vi "MasterAquisitionFile_2P.vi"() -> ()   [LabVIEW 2020]
uses:
  <vilib>/userDefined/High Color/IMAQdx.ctl
  <vilib>/vision/driver/IMAQdx.llb/IMAQdx Camera Control Mode.ctl
  <vilib>/vision/driver/IMAQdx.llb/IMAQdx Acquisition Mode.ctl
  <vilib>/vision/driver/IMAQdx.llb/IMAQdx Buffer Number Mode.ctl
  <vilib>/DAQmx/write.llb/DAQmx Write (Digital 1D Wfm NChan NSamp).vi
  <vilib>/DAQmx/read.llb/DAQmx Read (Digital 1D Bool 1Chan 1Samp).vi
  <vilib>/DAQmx/read.llb/DAQmx Read (Analog 1D Wfm NChan NSamp).vi
  <vilib>/Waveform/DWDTOps.llb/DWDT Digital to Boolean Array.vi
  <vilib>/DAQmx/create/channels.llb/DAQmx Create Channel (DO-Digital Output).vi
  <vilib>/DAQmx/configure/timing.llb/DAQmx Timing (Sample Clock).vi
  <vilib>/Waveform/DWDTOps.llb/DWDT Boolean Array to Digital.vi
  <vilib>/Waveform/DWDTOps.llb/DWDT Uncompress Digital.vi
  <vilib>/DAQmx/miscellaneous.llb/DAQmx Fill In Error Info.vi
  <vilib>/DAQmx/create/channels.llb/DAQmx Create Channel (DI-Digital Input).vi
  <vilib>/DAQmx/create/channels.llb/DAQmx Create Channel (CO-Pulse Generation-Frequency).vi
  <vilib>/DAQmx/configure/timing.llb/DAQmx Timing (Implicit).vi
  <vilib>/DAQmx/create/channels.llb/DAQmx Create Channel (AI-Voltage-Basic).vi
  <vilib>/DAQmx/configure/trigger.llb/DAQmx Start Trigger (Digital Edge).vi
  <vilib>/vision/driver/NI_Vision_Acquisition_Software.lvlib
  <resource>/objmgr/imaqdx.rc
  <resource>/objmgr/daqmx.rc
panel:
  out "Analog Data 3":bool
  out "?":T1(plugin-control)
  out "?":T1(plugin-control)
  out "Analog Data 2":bool
  in  "Pupil Fs":cluster{"Pupil Fs":u16}={"Pupil Fs"=30} {"Pupil Fs" format="%0.0f"}
  out "Pupil Cam Fs":dbl(knob) scale=0.0..200.0 scale format="%#1_6g"
  out "Dropped 2":u32(slide) caption="Pupil" scale=0.0..150.0
  out "Pupil Cam":bool
  in  "Analog Input Channels":tag="Dev1/ai0:3"
  out "Auditory":bool
  out "RPad":bool
  out "LPad":bool
  in  "Sol Stim Parameters":cluster{"Fs":dbl, "Samples":dbl}
  in  "LED Stim Parameters":cluster{"Fs":dbl, "Samples":dbl}
  in  "Generate Stimuli":bool
  in  "Sol Duty Cycle (%)":dbl=50.0
  in  "Sol Freq":dbl=5.0
  in  "Sol Dur (s)":dbl=5.0
  in  "LED Duty Cycle (%)":dbl=10.0
  in  "LED Freq":dbl=10.0
  in  "LED Dur (s)":dbl=2.0
  out "Stimulus Order":digitalwaveform[](graph)
  out "Solenoid Stim":digitalwaveform(graph)={"t0"=timestamp(0 s since 1904-01-01), "dt"=5e-05, "Y"={"transitions"=[], "data"=array100000x1[100000 elements]}}
  in  "Trial Offset (s)":dbl=45.0
  in  "Interstim (s)":dbl=45.0
  in  "Right Pad":dbl=1.0
  in  "Left Pad":dbl=1.0
  in  "Auditory":dbl=1.0
  in  "LED":dbl
  in  "stop":bool
  out "?":T1(plugin-control)
  out "Behavior Cam Fs":dbl(knob) scale=0.0..200.0
  out "Behav Cam":bool
  out "Complete":bool
  out "Whisk Cam":bool
  out "Analog":bool
  out "MScan Trig":bool
  out "?":bool[](array[boolean])=[TRUE]
  out "Hexadecimal Data":u32=1 format="%x"
  out "Time Elapsed (Min)":cluster{dbl, dbl}(slide)={1.0, 0.0} scale=0.0..16.0 scale format="%#_2g"
  out "Whisker Camera":bool
  out "Analog Data":bool
  out "Analog Samples":i32
  in  "Device Analog Channel Labels":string[](array[string])=["forceSensor", "LPadSol", "RPadSol", "AudSol", "", "", "", ""]
  in  "?":cluster{"Analog Fs":u16}={"Analog Fs"=20000} {"Analog Fs" format="%0.0f"}
  in  "?":cluster{"WhiskerCam Fs":u16}={"WhiskerCam Fs"=150}
  out "Notes Size":i32=7
  out "Notes Reversed":string[](array[string])=["Experimenter", "Animal ID", "Isoflurane time", "Amplifier Gain", "Session ID", "Hemisphere", "Solenoid PSI"]
  out "Notes Array":string[](array[string])=["Solenoid PSI", "Hemisphere", "Session ID", "Amplifier Gain", "Isoflurane time", "Animal ID", "Experimenter"]
  in  "Notes:":T2={"Experimenter"="Kevin\n", "Animal ID"="T300", "Isoflurane time"="730", "Amplifier Gain"="10000", "Session ID"="Imaging Session One", "Hemisphere"="RH", "Solenoid PSI"="10"}
  in  "Target Path":path=path "C:/Users/klt8/Documents" caption="Final Saved File Location"
  out "Dropped":u32(slide) caption="Whisk" scale=0.0..150.0
  out "Current File Name":string="221018_11_01_39"
  in  "Time (min)":dbl(knob)=1.0 min=0.5 max=20.0 step=0.5 scale=0.0..20.0 scale format="%#_3g"
  in  "Temp Path":path=path "C:/Users/klt8/Documents/LabVIEW Temp Files" caption="Temporary File Path"
  out "Whisker Cam Fs":dbl(knob) scale=0.0..200.0 scale format="%#1_6g"
  # "Notes"
  # "Dropped Frames"
  # "LPAD"
  # "RPAD"
  # "AUD"
  # "Analog Fs"
  # "Whisker Fs"
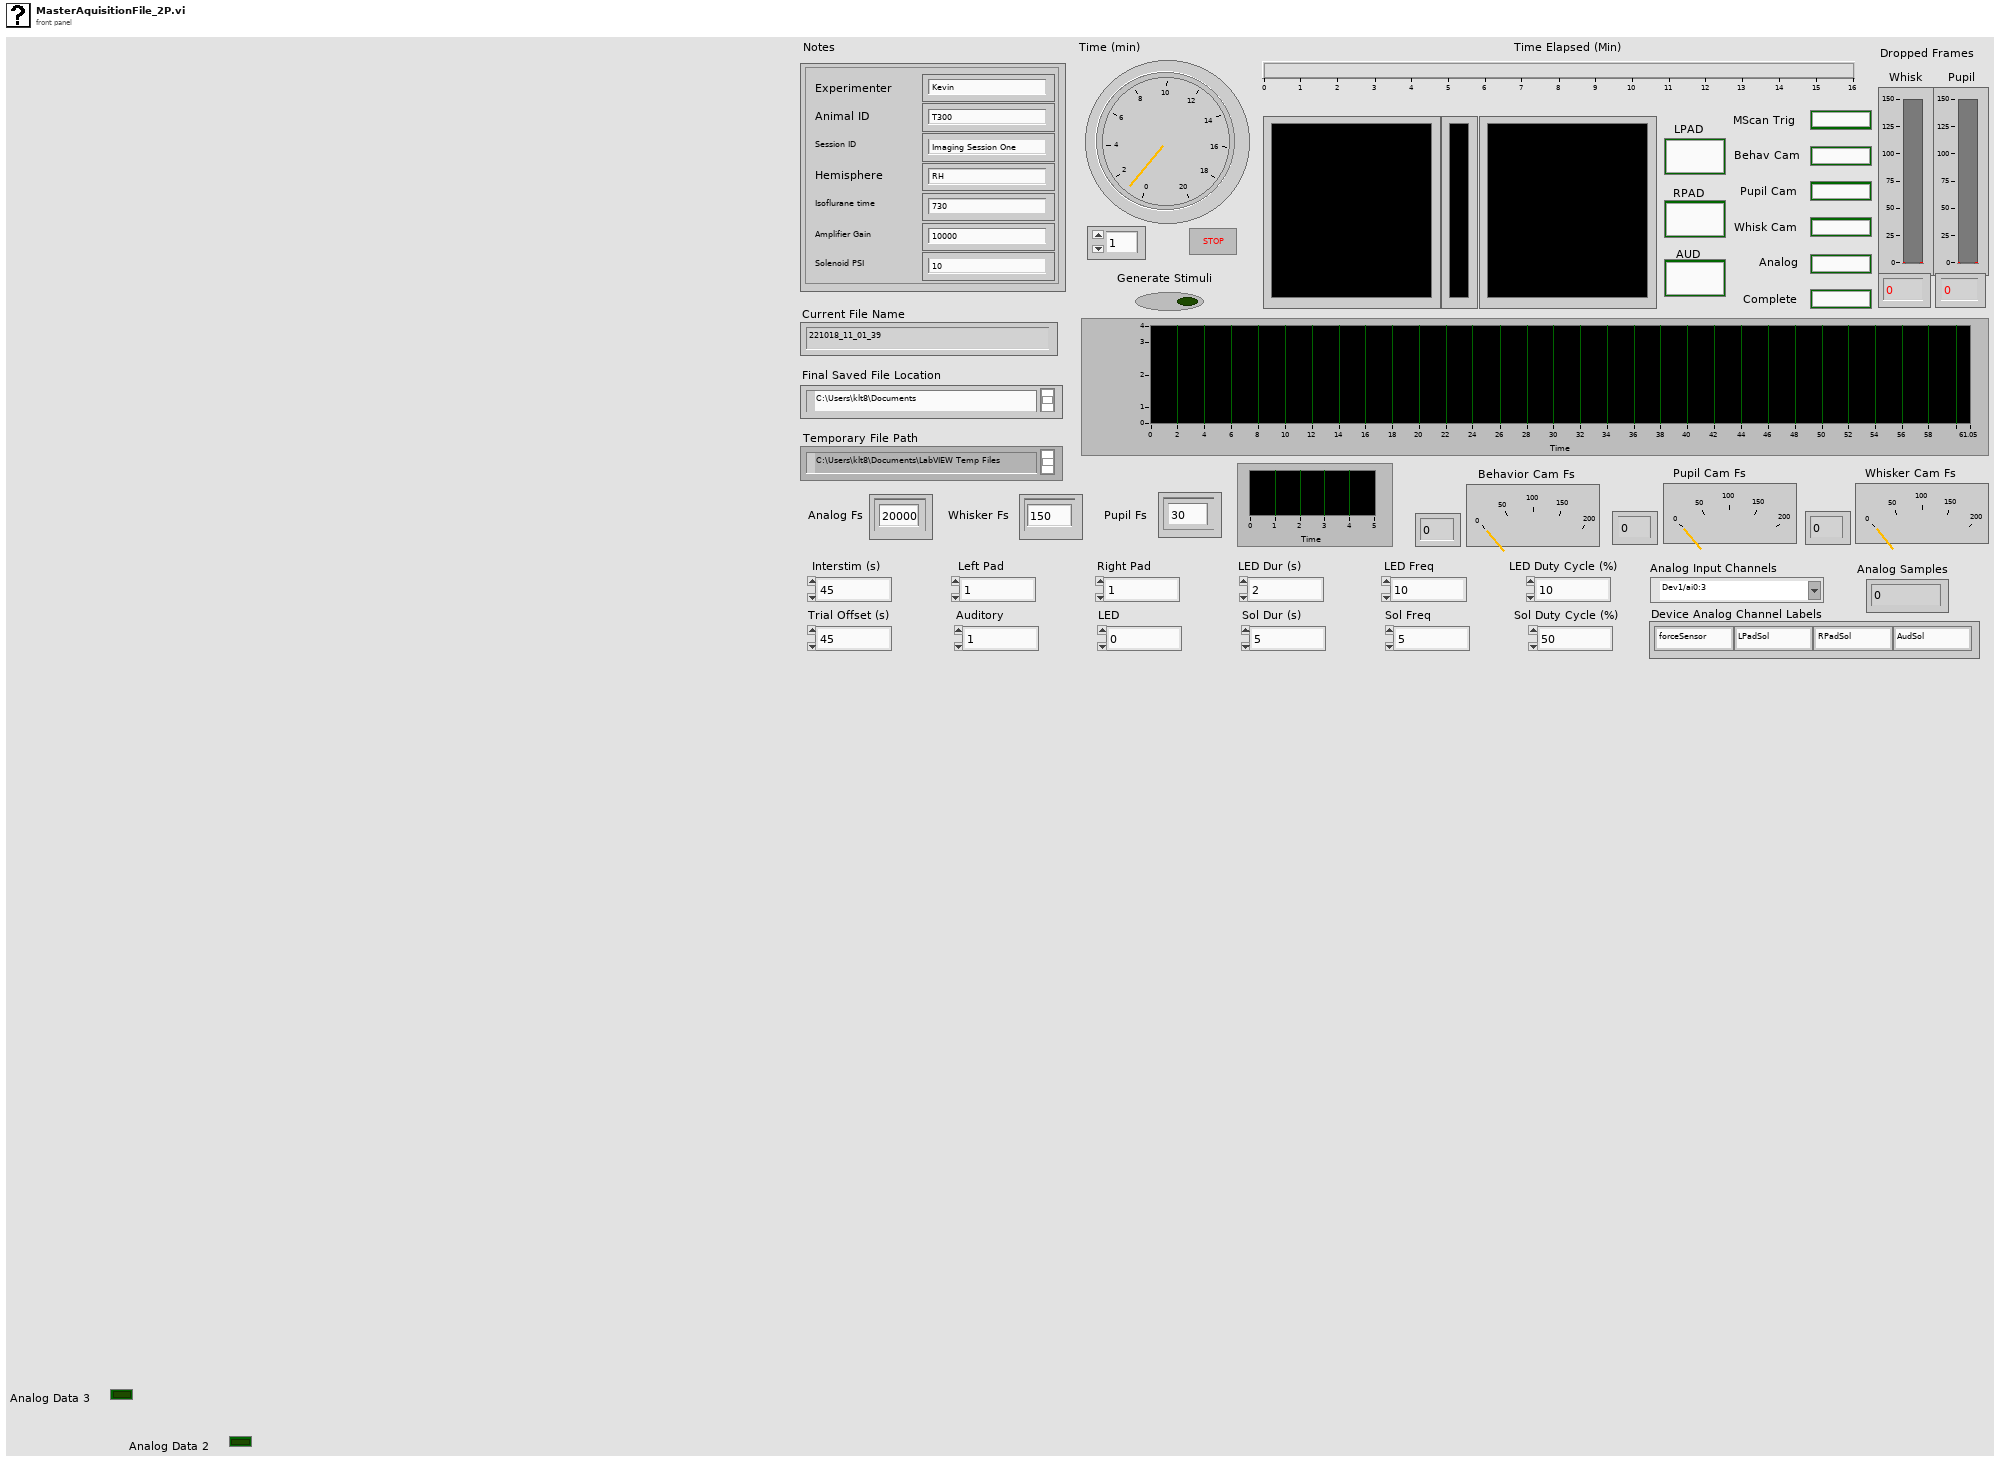
[diagram p1: front panel]
types:
  T1 = typedef "IMAQ Image.ctl" = refnum<image>
  T2 = cluster{"Experimenter":string, "Animal ID":string, "Isoflurane time":string, "Amplifier Gain":string, "Session ID":string, "Hemisphere":string, "Solenoid PSI":string}
  T3 = typedef "IMAQdx.ctl" = refnum<k21>
  T4 = enum16{"open", "replace", "create", "open or create", "replace or create", "replace or create with confirmation"}
  T5 = typedef "NI_Vision_Acquisition_Software.lvlib/IMAQdx Acquisition Mode.ctl" = enum32{"One Shot", "Continuous"}
  T6 = typedef "NI_Vision_Acquisition_Software.lvlib/IMAQdx Camera Control Mode.ctl" = enum32{"Controller", "Listener"}
  T7 = enum16{"open", "open or create", "create or replace", "create", "open (read-only)"}
  T8 = enum16{"big-endian, network order", "native, host order", "little-endian"}
  T9 = typedef "NI_Vision_Acquisition_Software.lvlib/IMAQdx Buffer Number Mode.ctl" = enum32{"Next", "Last", "Buffer Number", "Every", "Last New"}
  T10 = typedef "Image Type" = u32
  T11 = typedef "IMAQ AVI2 Refnum.ctl" = refnum<k20>
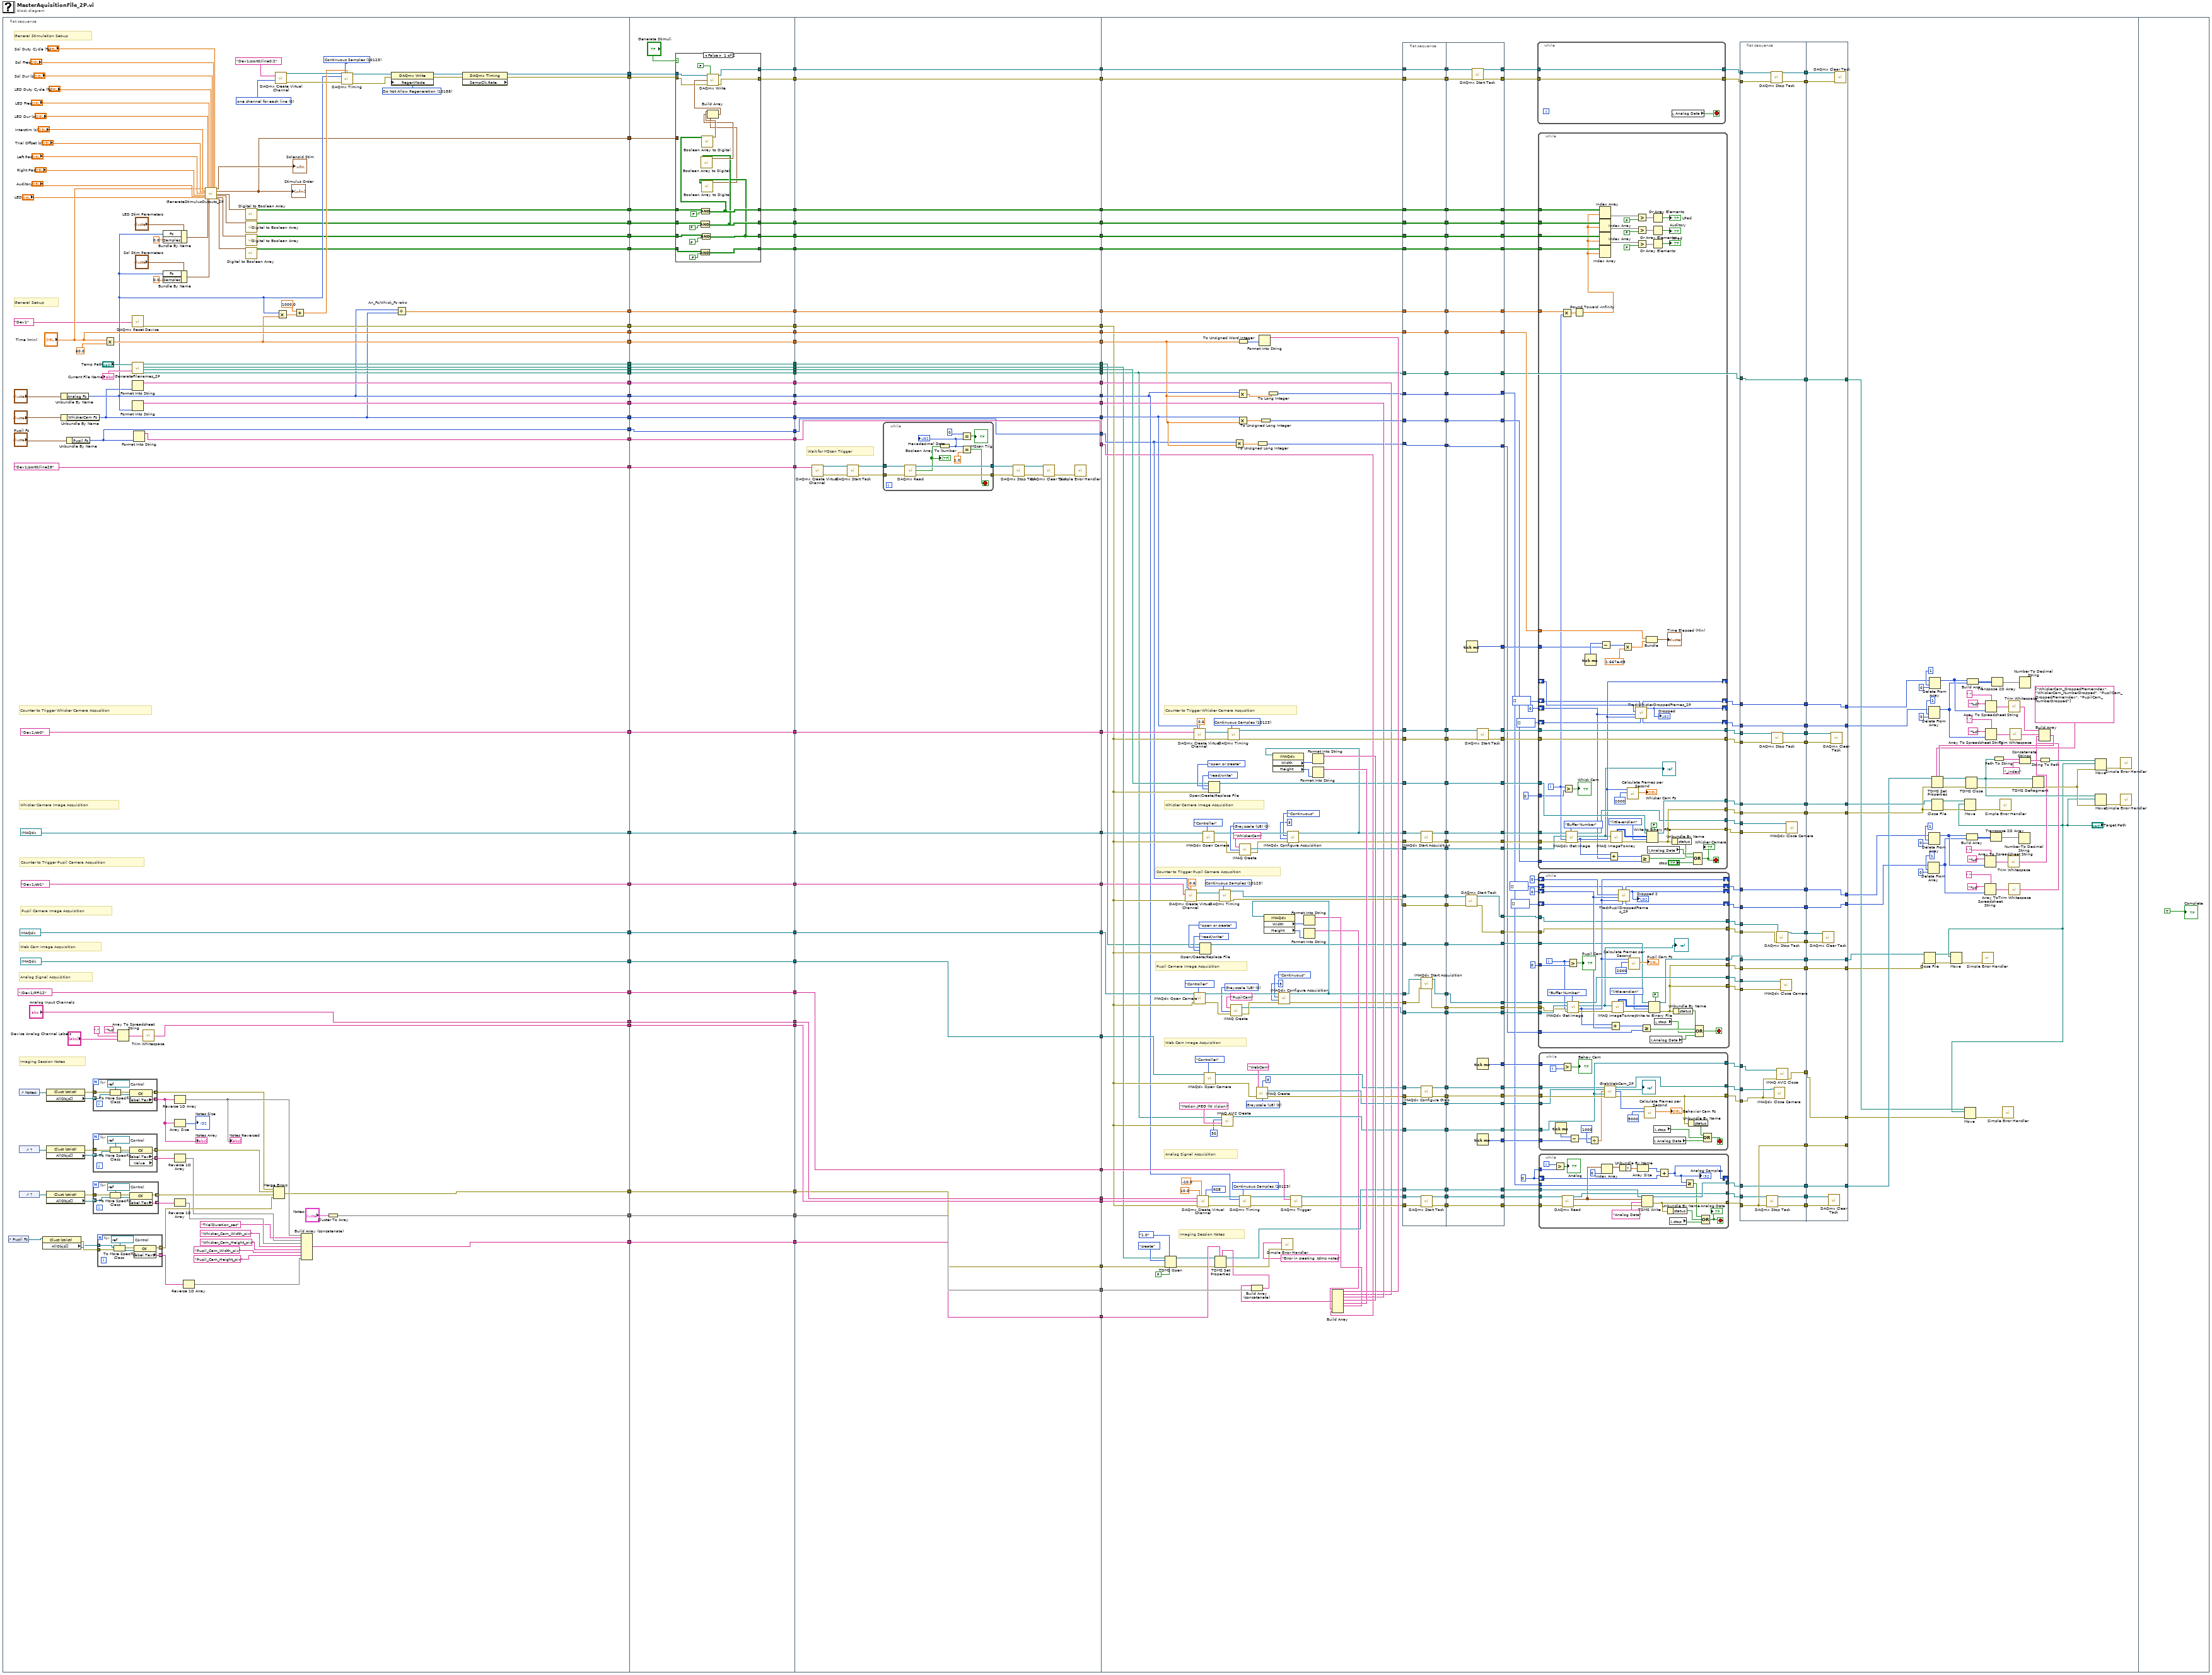
[diagram p0: block diagram]
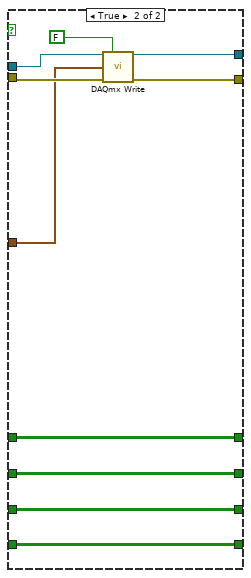
[diagram p2: hidden frame]
diagram:
  n1 = flat-sequence {
    tunnel: [tag "/Dev1/PFI12" ("Whisk Cam Trigger")] -> w70
    tunnel: [w131] -> w68
    tunnel: ["Time (min)"] -> w66
    tunnel: [w177] -> w64
    tunnel: [w176] -> w62
    tunnel: [w129] -> w60
    tunnel: [w128] -> w58
    tunnel: [w175] -> w56
    tunnel: [tag "Dev1/ctr0" ("Whisk Cam Counter")] -> w54
    tunnel: [w174] -> w52
    tunnel: ["Analog Input Channels"] -> w50
    tunnel: [T3 "cam2" ("Whisker Cam ID")] -> w48
    tunnel: [w173] -> w46
    tunnel: [w171] -> w44
    tunnel: [w172] -> w42
    tunnel: [T3 "cam1" ("WebCam ID")] -> w40
    tunnel: [tag "Dev1/port0/line28" ("MScan Trigger")] -> w38
    tunnel: [w168] -> w36
    tunnel: [w167] -> w34
    tunnel: [w166] -> w32
    tunnel: [w127] -> w24
    tunnel: [w117] -> w22
    tunnel: [w116] -> w21
    tunnel: [w115] -> w20
    tunnel: [w114] -> w19
    tunnel: [w113] -> w18
    tunnel: [w112] -> w17
    tunnel: [w111] -> w16
    tunnel: [tag "Dev1/ctr1" ("Whisk Cam Counter")] -> w15
    tunnel: [T3 "cam3" ("Whisker Cam ID")] -> w14
    tunnel: [w106] -> w9
    tunnel: [w105] -> w8
    tunnel: [w97] -> w1
    tunnel: w70 -> [w275]
    tunnel: [w275] -> w69
    tunnel: w68 -> [w274]
    tunnel: [w274] -> w67
    tunnel: w66 -> [w273]
    tunnel: [w273] -> w65
    tunnel: w64 -> [w272]
    tunnel: [w272] -> w63
    tunnel: w62 -> [w271]
    tunnel: [w271] -> w61
    tunnel: w60 -> [w270]
    tunnel: [w270] -> w59
    tunnel: w58 -> [w269]
    tunnel: [w269] -> w57
    tunnel: w56 -> [w268]
    tunnel: [w268] -> w55
    tunnel: w54 -> [w267]
    tunnel: [w267] -> w53
    tunnel: w52 -> [w266]
    tunnel: [w266] -> w51
    tunnel: w50 -> [w265]
    tunnel: [w265] -> w49
    tunnel: w48 -> [w264]
    tunnel: [w264] -> w47
    tunnel: w46 -> [w263]
    tunnel: [w263] -> w45
    tunnel: w44 -> [w262]
    tunnel: [w262] -> w43
    tunnel: w42 -> [w261]
    tunnel: [w261] -> w41
    tunnel: w40 -> [w260]
    tunnel: [w260] -> w39
    tunnel: w38 -> [w259]
    tunnel: [w259] -> w37
    tunnel: w36 -> [w258]
    tunnel: [w258] -> w35
    tunnel: w34 -> [w257]
    tunnel: [w257] -> w33
    tunnel: w32 -> [w256]
    tunnel: [w256] -> w31
    tunnel: [w247] -> w30
    tunnel: [w246] -> w29
    tunnel: [w245] -> w28
    tunnel: [w244] -> w27
    tunnel: [w243] -> w26
    tunnel: [w242] -> w25
    tunnel: w24 -> [w255]
    tunnel: [w255] -> w23
    tunnel: w22 -> [w254]
    tunnel: w21 -> [w253]
    tunnel: w20 -> [w252]
    tunnel: w19 -> [w251]
    tunnel: w18 -> [w250]
    tunnel: w17 -> [w249]
    tunnel: w16 -> [w248]
    tunnel: w15 -> [w239]
    tunnel: w14 -> [w240]
    tunnel: [w239] -> w13
    tunnel: [w240] -> w12
    tunnel: w9 -> [w237]
    tunnel: w8 -> [w238]
    tunnel: [w238] -> w7
    tunnel: [w237] -> w6
    tunnel: [w236] -> w2
    tunnel: w1 -> [w236]
    tunnel: [w324] -> w96
    tunnel: [w336] -> w95
    tunnel: [w337] -> w94
    tunnel: [w338] -> w93
    tunnel: [w339] -> w92
    tunnel: [w326] -> w91
    tunnel: [w340] -> w90
    tunnel: [w325] -> w89
    tunnel: [w341] -> w88
    tunnel: [w342] -> w87
    tunnel: [w343] -> w86
    tunnel: [w344] -> w85
    tunnel: [w345] -> w84
    tunnel: [w346] -> w83
    tunnel: [w347] -> w82
    tunnel: w69 -> [w347]
    tunnel: w67 -> [w346]
    tunnel: w65 -> [w345]
    tunnel: w63 -> [w344]
    tunnel: w61 -> [w343]
    tunnel: w59 -> [w342]
    tunnel: w57 -> [w341]
    tunnel: w55 -> [w325]
    tunnel: w53 -> [w340]
    tunnel: w51 -> [w326]
    tunnel: w49 -> [w339]
    tunnel: w47 -> [w338]
    tunnel: w45 -> [w337]
    tunnel: w43 -> [w336]
    tunnel: w41 -> [w324]
    tunnel: [w322] -> w81
    tunnel: w39 -> [w322]
    tunnel: w37 -> [w323]
    tunnel: w35 -> [w321]
    tunnel: [w321] -> w80
    tunnel: w33 -> [w320]
    tunnel: w31 -> [w319]
    tunnel: [w320] -> w79
    tunnel: [w319] -> w78
    tunnel: [w318] -> w77
    tunnel: w30 -> [w318]
    tunnel: [w317] -> w76
    tunnel: w29 -> [w317]
    tunnel: [w316] -> w75
    tunnel: w28 -> [w316]
    tunnel: [w315] -> w74
    tunnel: w27 -> [w315]
    tunnel: [w314] -> w73
    tunnel: w26 -> [w314]
    tunnel: w25 -> [w313]
    tunnel: [w313] -> w72
    tunnel: [w312] -> w71
    tunnel: w23 -> [w312]
    tunnel: w13 -> [w310]
    tunnel: w12 -> [w311]
    tunnel: [w310] -> w11
    tunnel: [w311] -> w10
    tunnel: w7 -> [w308]
    tunnel: w6 -> [w309]
    tunnel: [w309] -> w5
    tunnel: [w308] -> w4
    tunnel: [w307] -> w3
    tunnel: w2 -> [w307]
    tunnel: w96 -> [w562]
    tunnel: w95 -> [w570]
    tunnel: w94 -> [w459]
    tunnel: w93 -> [w569]
    tunnel: w92 -> [w568]
    tunnel: w91 -> [w567]
    tunnel: w90 -> [w566]
    tunnel: w89 -> [w565]
    tunnel: w88 -> [w536]
    tunnel: w87 -> [w387]
    tunnel: w86 -> [w564]
    tunnel: w85 -> [w526]
    tunnel: w84 -> [w559]
    tunnel: w83 -> [w388]
    tunnel: w82 -> [w563]
    tunnel: w81 -> [w550]
    tunnel: w80 -> [w370]
    tunnel: w79 -> [w532]
    tunnel: w78 -> [w530]
    tunnel: w77 -> [w489]
    tunnel: w76 -> [w487]
    tunnel: w75 -> [w493]
    tunnel: w74 -> [w492]
    tunnel: w73 -> [w491]
    tunnel: w72 -> [w490]
    tunnel: w71 -> [w509]
    tunnel: w11 -> [w425]
    tunnel: w10 -> [w461]
    tunnel: w5 -> [w385]
    tunnel: w4 -> [w386]
    tunnel: w3 -> [w383]
    frame #0 {
      w146 = 10158 items=["Allow Regeneration"=10097, "Do Not Allow Regeneration"=10158] ("RegenMode")
      w147 = 10123 items=["Finite Samples"=10178, "Continuous Samples"=10123, "Hardware Timed Single Point"=12522] ("sample mode")
      w150 = 0 items=["one channel for each line", "one channel for all lines"] ("line grouping")
      # "Counter to Trigger Pupil Camera Acqusition"
      # "Pupil Camera Image Acquisition"
      # "General Stimulation Set-up"
      # "General Set-up"
      # "Whisker Camera Image Acquisition"
      # "Imaging Session Notes"
      # "Counter to Trigger Whisker Camera Acqusition"
      # "Web Cam Image Acquisition"
      # "Analog Signal Acquisition"
      n2 = control-ref of="Pupil Fs"() -> (w104:refnum<vi>)
      n3 = control-ref of="Notes:"() -> (w193:refnum<vi>)
      n4 = control-ref of="?"() -> (w191:refnum<vi>)
      n5 = control-ref of="?"() -> (w184:refnum<vi>)
      n6 = property class="Clust (strict)"(reference=w104) -> (error out=w102:errorcluster, "AllObjs[]"=w101:refnum<vi>[])  [unwired: 1 in, 1 out]
      n7 = property class="Clust (strict)"(reference=w193) -> (error out=w192:errorcluster, "AllObjs[]"=w194:refnum<vi>[])  [unwired: 1 in, 1 out]
      n8 = property class="Clust (strict)"(reference=w191) -> (error out=w189:errorcluster, "AllObjs[]"=w190:refnum<vi>[])  [unwired: 1 in, 1 out]
      n9 = property class="Clust (strict)"(reference=w184) -> (error out=w185:errorcluster, "AllObjs[]"=w187:refnum<vi>[])  [unwired: 1 in, 1 out]
      n10 = Unbundle By Name("?") -> ("Analog Fs"=w129:u16)
      n11 = Unbundle By Name("?") -> ("WhiskerCam Fs"=w128:u16)
      n12 = Unbundle By Name("Pupil Fs") -> ("Pupil Fs"=w105:u16)
      n13 = for {
        tunnel: [w219] -> w199 mode=indexing
        tunnel: w194 -> [w218] mode=indexing
        tunnel: w192 -> [w217]
        tunnel: [w215] -> w198 mode=indexing
        w220 = refnum<vi> refnum  # Control
        n14 = To More Specific Class(target class=w220, reference=w218, error in=w217) -> (specific class reference=w221:refnum<vi>, error out=w216:errorcluster)
        n15 = property class="Ctl"(reference=w221, error in=w216) -> (error out=w215:errorcluster, "Label.Text"=w219:string)  [unwired: 1 out]
      }
      "Notes Array" <- w199
      n16 = for {
        tunnel: [w226] -> w188 mode=indexing
        tunnel: w190 -> [w225] mode=indexing
        tunnel: w189 -> [w224]
        tunnel: [w222] -> w197 mode=indexing
        w227 = refnum<vi> refnum  # Control
        n17 = To More Specific Class(target class=w227, reference=w225, error in=w224) -> (specific class reference=w228:refnum<vi>, error out=w223:errorcluster)
        n18 = property class="Ctl" props=["Label", "Text", "Value"](reference=w228, error in=w223) -> (error out=w222:errorcluster, "Label.Text"=w226:string)  [unwired: 2 out]
      }
      n19 = for {
        tunnel: [w233] -> w186 mode=indexing
        tunnel: w187 -> [w232] mode=indexing
        tunnel: w185 -> [w231]
        tunnel: [w229] -> w196 mode=indexing
        w234 = refnum<vi> refnum  # Control
        n20 = To More Specific Class(target class=w234, reference=w232, error in=w231) -> (specific class reference=w235:refnum<vi>, error out=w230:errorcluster)
        n21 = property class="Ctl"(reference=w235, error in=w230) -> (error out=w229:errorcluster, "Label.Text"=w233:string)  [unwired: 1 out]
      }
      n22 = for {
        tunnel: [w212] -> w99 mode=indexing
        tunnel: [w210] -> w100 mode=indexing
        tunnel: w102 -> [w209]
        tunnel: w101 -> [w208] mode=indexing
        w213 = refnum<vi> refnum  # Control
        n23 = To More Specific Class(target class=w213, reference=w208, error in=w209) -> (specific class reference=w214:refnum<vi>, error out=w211:errorcluster)
        n24 = property class="Ctl"(reference=w214, error in=w211) -> (error out=w210:errorcluster, "Label.Text"=w212:string)  [unwired: 1 out]
      }
      n25 = Multiply(x="Time (min)", y=60.0) -> (x*y=w131:dbl)
      n26 = Array To Spreadsheet String(delimiter (Tab)=",", array="Device Analog Channel Labels", 3:"%s" ("format string")) -> (spreadsheet string=w201:string)
      n27 = call <vilib>:"DAQmx Reset Device.vi"("device in"=tag "Dev1" ("NI Board")) -> ("error out"=w173:errorcluster)  [unwired: 14 in]
      n28 = call "GenerateFilenames_2P.vi"("path"="Temp Path") -> ("Analog file name"=→"Current File Name":string, "Pupil Path"=w97:path, "TDMS Path"=w166:path, "Whisker Path"=w171:path, "WebCam Path"=w168:path)
      n29 = Format Into String(w128) -> (resulting string=w177:string)  [unwired: 3 in, 1 out]
      n30 = Format Into String(w129) -> (resulting string=w176:string)  [unwired: 3 in, 1 out]
      n31 = Format Into String(w105) -> (resulting string=w106:string)  [unwired: 3 in, 1 out]
      n32 = call <vilib>:"Trim Whitespace.vi"("string"=w201) -> ("trimmed string"=w174:string)  [unwired: 1 in]
      n33 = Bundle By Name(cluster="LED Stim Parameters", "Fs"=w129, "Samples"=0.0) -> (w136:cluster{"Fs":dbl, "Samples":dbl})
      n34 = Bundle By Name(cluster="Sol Stim Parameters", "Fs"=w129, "Samples"=0.0) -> (w135:cluster{"Fs":dbl, "Samples":dbl})
      n35 = Reverse 1D Array(array=w199) -> (reversed array=w200:string[])
      "Notes Reversed" <- w200
      n36 = Array Size(array=w199) -> (size(s)=→"Notes Size":i32)
      n37 = Reverse 1D Array(array=w188) -> (reversed array=w206:string[])
      n38 = Reverse 1D Array(array=w186) -> (reversed array=w207:string[])
      n39 = Reverse 1D Array(array=w99) -> (reversed array=w98:string[])
      n40 = call "GenerateStimulusOutputs_2P.vi"("Trial duration (min)"="Time (min)", "Rest duration(s)"="Interstim (s)", "trial offset (s)"="Trial Offset (s)", "Left Pad"="Left Pad", "Right Pad"="Right Pad", "Auditory"="Auditory", "LED"="LED", "LED Stim Duration (s)"="LED Dur (s)", "LED Stim Parameters"=w136, "LED Frequency"="LED Freq", "Sol Stim Parameters"=w135, "LED duty cycle (%)"="LED Duty Cycle (%)", "Sol Stim Duration (s)"="Sol Dur (s)", "Sol Frequency"="Sol Freq", "Sol Duty Cycle (%)"="Sol Duty Cycle (%)") -> ("Solenoid Stim Waveforms"=→"Solenoid Stim":digitalwaveform, "Stimulus Digital Outputs"=w113:digitalwaveform[], "Left Pad Out"=w125:digitalwaveform, "Auditory Out"=w152:digitalwaveform, "Right Pad Out"=w151:digitalwaveform, "LED Out"=w130:digitalwaveform)  [unwired: 7 in]
      "Stimulus Order" <- w113
      n41 = call-poly <vilib>:"Digital to Boolean Array.vi"("digital waveform"=w125) -> ("boolean array"=w112:bool[][])  [unwired: 9 in, 1 out]
      n42 = call-poly <vilib>:"Digital to Boolean Array.vi"("digital waveform"=w152) -> ("boolean array"=w115:bool[][])  [unwired: 9 in, 1 out]
      n43 = call-poly <vilib>:"Digital to Boolean Array.vi"("digital waveform"=w151) -> ("boolean array"=w114:bool[][])  [unwired: 9 in, 1 out]
      n44 = call-poly <vilib>:"Digital to Boolean Array.vi"("digital waveform"=w130) -> ("boolean array"=w111:bool[][])  [unwired: 9 in, 1 out]
      n45 = Merge Errors(w198, w197, w196, w100) -> (w167:errorcluster)
      n46 = call-poly <vilib>:"DAQmx Create Virtual Channel.vi"("lines"=tag "Dev1/port0/line0:2", "line grouping"=w150) -> ("task out"=w149:refnum<k21>, "error out"=w148:errorcluster)  [unwired: 12 in]
      n47 = Multiply(x=w129, y=w131) -> (x*y=w134:dbl)
      n48 = Add(x=1000.0, y=w134) -> (x+y=w132:dbl)
      n49 = Build Array (concatenate)(w200, "TrialDuration_sec", w206, w207, "Whisker_Cam_Width_pix", "Whisker_Cam_Height_pix", "Pupil_Cam_Width_pix", "Pupil_Cam_Height_pix", w98) -> (w172:string[])
      n50 = Cluster To Array(cluster="Notes:") -> (array=w175:string[])
      n51 = call-poly <vilib>:"DAQmx Timing.vi"("task/channels in"=w149, "sample mode"=w147, "samples per channel"=w132, "rate"=w129, "error in"=w148) -> ("task out"=w143:refnum<k21>, "error out"=w142:errorcluster)  [unwired: 9 in]
      n52 = property class="DAQmx Write"(reference=w143, error in=w142, "RegenMode"=w146) -> (reference out=w144:refnum<k21>, error out=w145:errorcluster)
      n53 = Divide "An_Fs/Whisk_Fs ratio"(x=w129, y=w128) -> (x/y=w127:dbl)
      n54 = property class="DAQmx Timing" props=["SampClk.Rate"](reference=w144, error in=w145) -> (reference out=w117:refnum<k21>, error out=w116:errorcluster)  [unwired: 1 out]
    }
    frame #1 {
      n55 = case shown="False" "Generate Stimuli" {
        tunnel: w254 -> [w283 w306]
        tunnel: w253 -> [w282 w305]
        tunnel: [w280 w304] -> w247
        tunnel: [w281 w303] -> w246
        tunnel: w252 -> [w295 w302]
        tunnel: w251 -> [w296 w301]
        tunnel: [w279 w299] -> w245
        tunnel: [w278 w302] -> w244
        tunnel: [w277 w301] -> w243
        tunnel: [w289 w298] -> w242
        tunnel: w250 -> [_ w300]
        tunnel: w249 -> [w290 w299]
        tunnel: w248 -> [w288 w298]
        frame False {
          n56 = Compound Arithmetic op=AND(w295, FALSE) -> (w278:bool[][])
          n57 = call-poly <vilib>:"Boolean Array to Digital.vi"("boolean array"=w278) -> ("digital waveform"=w285:digitalwaveform)  [unwired: 9 in, 1 out]
          n58 = Compound Arithmetic op=AND(w288, FALSE) -> (w289:bool[][])
          n59 = Compound Arithmetic op=AND(w290, FALSE) -> (w279:bool[][])
          n60 = call-poly <vilib>:"Boolean Array to Digital.vi"("boolean array"=w279) -> ("digital waveform"=w286:digitalwaveform)  [unwired: 9 in, 1 out]
          n61 = Compound Arithmetic op=AND(w296, FALSE) -> (w277:bool[][])
          n62 = call-poly <vilib>:"Boolean Array to Digital.vi"("boolean array"=w277) -> ("digital waveform"=w276:digitalwaveform)  [unwired: 9 in, 1 out]
          n63 = Build Array(w286, w285, w276) -> (w284:digitalwaveform[])
          n64 = call-poly <vilib>:"DAQmx Write.vi"("task/channels in"=w283, "auto start"=FALSE, "data"=w284, "error in"=w282) -> ("task out"=w280:refnum<k21>, "error out"=w281:errorcluster)  [unwired: 9 in, 1 out]
        }
        frame True {
          n65 = call-poly <vilib>:"DAQmx Write.vi"("task/channels in"=w306, "auto start"=FALSE, "data"=w300, "error in"=w305) -> ("task out"=w304:refnum<k21>, "error out"=w303:errorcluster)  [unwired: 9 in, 1 out]
        }
      }
    }
    frame #2 {
      # "Wait for MScan Trigger"
      n66 = call-poly <vilib>:"DAQmx Create Virtual Channel.vi"("lines"=w323) -> ("task out"=w331:refnum<k21>, "error out"=w332:errorcluster)  [unwired: 13 in]
      n67 = call <vilib>:"DAQmx Start Task.vi"("task/channels in"=w331, "error in"=w332) -> ("task out"=w335:refnum<k21>, "error out"=w334:errorcluster)  [unwired: 12 in]
      n68 = while {
        tunnel: w335 -> [w357]
        tunnel: w334 -> [w356]
        tunnel: [w354] -> w329
        tunnel: [w355] -> w330
        stop <- w349 stop-if-true
        n69 = call-poly <vilib>:"DAQmx Read.vi"("task/channels in"=w357, "error in"=w356) -> ("task out"=w355:refnum<k21>, "data"=w353:bool[], "error out"=w354:errorcluster)  [unwired: 11 in]
        "?" <- w353
        n70 = Boolean Array To Number(Boolean array=w353) -> (number=w348:u32)
        "Hexadecimal Data" <- w348
        n71 = Equal?(x=w348, y=u32 0) -> (x = y?=→"MScan Trig":bool)
        n72 = Equal?(x=w348, y=1.0) -> (x = y?=w349:bool)
      }
      n73 = call <vilib>:"DAQmx Stop Task.vi"("task/channels in"=w330, "error in"=w329) -> ("task out"=w328:refnum<k21>, "error out"=w327:errorcluster)  [unwired: 12 in]
      n74 = call <vilib>:"DAQmx Clear Task.vi"("task in"=w328, "error in"=w327) -> ("error out"=w333:errorcluster)  [unwired: 13 in]
      n75 = call <vilib>:"Simple Error Handler.vi"("error in (no error)"=w333) -> ()  [unwired: 4 in, 5 out]
    }
    frame #3 {
      w463 = 10123 items=["Finite Samples"=10178, "Continuous Samples"=10123, "Hardware Timed Single Point"=12522] ("sample mode")
      w462 = T10 0 items=["Grayscale (U8)", "Grayscale (I16)", "Grayscale (SGL)", "Complex (CSG)", "RGB (U32)", "HSL (U32)", "RGB (U64)", "Grayscale (U16)"] ("Image Type")
      w554 = T10 0 items=["Grayscale (U8)", "Grayscale (I16)", "Grayscale (SGL)", "Complex (CSG)", "RGB (U32)", "HSL (U32)", "RGB (U64)", "Grayscale (U16)"] ("Image Type")
      w478 = u32 0 ("y")
      w579 = 10123 items=["Finite Samples"=10178, "Continuous Samples"=10123, "Hardware Timed Single Point"=12522] ("sample mode")
      w578 = 10083 items=["default"=-1, "RSE"=10083, "NRSE"=10078, "Differential"=10106, "Pseudodifferential"=12529] ("input terminal configuration")
      w580 = 10123 items=["Finite Samples"=10178, "Continuous Samples"=10123, "Hardware Timed Single Point"=12522] ("sample mode")
      w576 = T10 0 items=["Grayscale (U8)", "Grayscale (I16)", "Grayscale (SGL)", "Complex (CSG)", "RGB (U32)", "HSL (U32)", "RGB (U64)", "Grayscale (U16)"] ("Image Type")
      # "Pupil Camera Image Acquisition"
      # "Counter to Trigger Pupil Camera Acqusition"
      # "Whisker Camera Image Acquisition"
      # "Imaging Session Notes"
      # "Counter to Trigger Whisker Camera Acqusition"
      # "Web Cam Image Acquisition"
      # "Analog Signal Acquisition"
      n76 = TDMS Open(6:FALSE ("disable buffering? (T)"), 7:enum16{"1.0", "2.0"}."1.0" ("file format version (2.0)"), 8:w532, 10:T7."create" ("operation (0:open)"), 11:w530) -> (0:w529:errorcluster, 3:w528:refnum<k34>)  [unwired: 2 in]
      n77 = call-poly <vilib>:"DAQmx Create Virtual Channel.vi"("frequency"=w386, "duty cycle"=0.6, "counter"=w425, "error in"=w459) -> ("task out"=w474:refnum<k21>, "error out"=w475:errorcluster)  [unwired: 10 in]
      n78 = call-poly <vilib>:"DAQmx Create Virtual Channel.vi"("frequency"=w536, "duty cycle"=0.6, "counter"=w566, "error in"=w459) -> ("task out"=w601:refnum<k21>, "error out"=w602:errorcluster)  [unwired: 10 in]
      n79 = call <vilib>:"IMAQdx Open Camera.vi"("Camera Control Mode"=IMAQdx_Camera_Control_Mode."Controller", "error in"=w459, "Session In"=w461) -> ("error out"=w472:errorcluster, "Session Out"=w471:T3)  [unwired: 7 in]
      n80 = call-poly <vilib>:"DAQmx Create Virtual Channel.vi"("maximum value"=10.0, "minimum value"=-10.0, "input terminal configuration"=w578, "physical channels"=w568, "name to assign"=w567, "error in"=w459) -> ("task out"=w609:refnum<k21>, "error out"=w610:errorcluster)  [unwired: 8 in]
      n81 = Open/Create/Replace File(file path (use dialog)=w383, error in=w459, operation (0:open)=T4."open or create", access (0:read/write)=enum16{"read/write", "read-only", "write-only"}."read/write") -> (refnum out=w458:refnum<file>)  [unwired: 2 in, 2 out]
      n82 = call <vilib>:"IMAQdx Open Camera.vi"("Camera Control Mode"=IMAQdx_Camera_Control_Mode."Controller", "error in"=w459, "Session In"=w569) -> ("error out"=w599:errorcluster, "Session Out"=w598:T3)  [unwired: 7 in]
      n83 = call <vilib>:"IMAQdx Open Camera.vi"("Camera Control Mode"=IMAQdx_Camera_Control_Mode."Controller", "error in"=w459, "Session In"=w550) -> ("error out"=w551:errorcluster, "Session Out"=w549:T3)  [unwired: 7 in]
      n84 = Open/Create/Replace File(file path (use dialog)=w570, error in=w459, operation (0:open)=T4."open or create", access (0:read/write)=enum16{"read/write", "read-only", "write-only"}."read/write") -> (refnum out=w608:refnum<file>)  [unwired: 2 in, 2 out]
      n85 = call-poly <vilib>:"DAQmx Timing.vi"("task/channels in"=w474, "sample mode"=w463, "error in"=w475) -> ("task out"=w401:refnum<k21>, "error out"=w399:errorcluster)  [unwired: 11 in]
      n86 = call "IMAQ AVI2 Create"("error in (no error)"=w459, "Codec"="Motion JPEG (NI Vision)", "Frames Per Second"=u32 30, "AVI Path"=w370) -> ("AVI Refnum"=w538:T11)  [unwired: 6 in, 1 out]
      n87 = call-poly <vilib>:"DAQmx Timing.vi"("task/channels in"=w601, "sample mode"=w580, "error in"=w602) -> ("task out"=w618:refnum<k21>, "error out"=w619:errorcluster)  [unwired: 11 in]
      n88 = call "IMAQ Create"("Image Name"="PupilCam", "Image Type"=w462, "error in (no error)"=w472) -> ("New Image"=w408:T1, "error out"=w473:errorcluster)  [unwired: 2 in]
      n89 = Multiply(x=w386, y=w388) -> (x*y=w393:dbl)
      n90 = Multiply(x=w387, y=w388) -> (x*y=w390:dbl)
      n91 = Multiply(x=w536, y=w388) -> (x*y=w641:dbl)
      n92 = To Unsigned Word Integer(number=w388) -> (unsigned 16bit integer=w631:u16)
      n93 = call "IMAQ Create"("Image Name"="WhiskerCam", "Image Type"=w576, "error in (no error)"=w599) -> ("New Image"=w634:T1, "error out"=w600:errorcluster)  [unwired: 2 in]
      n94 = call-poly <vilib>:"DAQmx Timing.vi"("task/channels in"=w609, "sample mode"=w579, "rate"=w387, "error in"=w610) -> ("task out"=w611:refnum<k21>, "error out"=w612:errorcluster)  [unwired: 10 in]
      n95 = call "IMAQ Create"("Border Size"=3, "Image Name"="WebCam", "Image Type"=w554, "error in (no error)"=w551) -> ("New Image"=w547:T1, "error out"=w548:errorcluster)  [unwired: 1 in]
      n96 = To Unsigned Long Integer(number=w393) -> (unsigned 32bit integer=w391:u32)
      n97 = Format Into String(w631) -> (resulting string=w647:string)  [unwired: 3 in, 1 out]
      n98 = To Unsigned Long Integer(number=w641) -> (unsigned 32bit integer=w642:u32)
      n99 = To Long Integer(number=w390) -> (32bit integer=w389:i32)
      n100 = call <vilib>:"IMAQdx Configure Acquisition.vi"("error in"=w473, "Number of Buffers"=u32 5, "Continuous?"=IMAQdx_Acquisition_Mode."Continuous", "Session In"=w471) -> ("error out"=w405:errorcluster, "Session Out"=w460:T3)  [unwired: 6 in]
      n101 = property class="IMAQdx"(reference=w460) -> ("Width"=w476:u32, "Height"=w477:u32)  [unwired: 1 in, 2 out]
      n102 = call <vilib>:"IMAQdx Configure Acquisition.vi"("error in"=w600, "Number of Buffers"=u32 5, "Continuous?"=IMAQdx_Acquisition_Mode."Continuous", "Session In"=w598) -> ("error out"=w603:errorcluster, "Session Out"=w527:T3)  [unwired: 6 in]
      n103 = property class="IMAQdx"(reference=w527) -> ("Width"=w632:u32, "Height"=w633:u32)  [unwired: 1 in, 2 out]
      n104 = call-poly <vilib>:"DAQmx Trigger.vi"("task/channels in"=w611, "source"=w563, "error in"=w612) -> ("task out"=w613:refnum<k21>, "error out"=w614:errorcluster)  [unwired: 11 in]
      n105 = Format Into String(w476) -> (resulting string=w424:string)  [unwired: 3 in, 1 out]
      n106 = Format Into String(w477) -> (resulting string=w423:string)  [unwired: 3 in, 1 out]
      n107 = Format Into String(w632) -> (resulting string=w646:string)  [unwired: 3 in, 1 out]
      n108 = Format Into String(w633) -> (resulting string=w645:string)  [unwired: 3 in, 1 out]
      n109 = Build Array(w647, w526, w564, w646, w645, w424, w423, w385) -> (w524:string[])
      n110 = Build Array (concatenate)(w565, w524) -> (w571:string[])
      n111 = TDMS Set Properties(5:w571, 7:w562, 8:w529, 11:w528) -> (0:w630:errorcluster, 3:w629:refnum<k34>)  [unwired: 2 in, 2 out]
      n112 = call <vilib>:"Simple Error Handler.vi"("error source (\" \")"="Error in creating .tdms notes" ("error source (\" \")"), "error in (no error)"=w630) -> ()  [unwired: 3 in, 5 out]
      n113 = flat-sequence {
        tunnel: w527 -> [w835]
        tunnel: w603 -> [w834]
        tunnel: [w833] -> w658
        tunnel: [w832] -> w657
        tunnel: [w831] -> w656
        tunnel: w634 -> [w831]
        tunnel: [w830] -> w655
        tunnel: w608 -> [w830]
        tunnel: w613 -> [w829]
        tunnel: w614 -> [w828]
        tunnel: [w827] -> w654
        tunnel: [w826] -> w653
        tunnel: [w825] -> w652
        tunnel: w629 -> [w825]
        tunnel: w618 -> [w824]
        tunnel: [w824] -> w651
        tunnel: w619 -> [w823]
        tunnel: [w823] -> w650
        tunnel: w389 -> [w822]
        tunnel: [w822] -> w649
        tunnel: w642 -> [w821]
        tunnel: [w821] -> w648
        tunnel: w559 -> [w820]
        tunnel: [w820] -> w558
        tunnel: w549 -> [w819]
        tunnel: w548 -> [w818]
        tunnel: w547 -> [w817]
        tunnel: [w817] -> w546
        tunnel: [w816] -> w545
        tunnel: [w815] -> w544
        tunnel: [w814] -> w539
        tunnel: w538 -> [w814]
        tunnel: [w813] -> w518
        tunnel: w493 -> [w813]
        tunnel: [w812] -> w517
        tunnel: w492 -> [w812]
        tunnel: [w811] -> w516
        tunnel: w491 -> [w811]
        tunnel: [w810] -> w515
        tunnel: w490 -> [w810]
        tunnel: [w809] -> w510
        tunnel: w509 -> [w809]
        tunnel: w489 -> [w807]
        tunnel: [w808] -> w488
        tunnel: w487 -> [w808]
        tunnel: [w807] -> w486
        tunnel: w460 -> [w801]
        tunnel: w458 -> [w806]
        tunnel: [w806] -> w457
        tunnel: [w800] -> w411
        tunnel: w408 -> [w805]
        tunnel: [w805] -> w407
        tunnel: w405 -> [w799]
        tunnel: [w798] -> w404
        tunnel: [w804] -> w402
        tunnel: w401 -> [w804]
        tunnel: w399 -> [w803]
        tunnel: [w803] -> w398
        tunnel: [w802] -> w392
        tunnel: w391 -> [w802]
        tunnel: w370 -> [w797]
        tunnel: [w797] -> w373
        tunnel: [w868] -> w560
        tunnel: [w867] -> w561
        tunnel: [w875] -> w604
        tunnel: w658 -> [w875]
        tunnel: [w874] -> w605
        tunnel: w657 -> [w874]
        tunnel: [w873] -> w606
        tunnel: w656 -> [w873]
        tunnel: [w872] -> w607
        tunnel: w655 -> [w872]
        tunnel: [w871] -> w616
        tunnel: w654 -> [w871]
        tunnel: [w870] -> w615
        tunnel: w653 -> [w870]
        tunnel: [w869] -> w617
        tunnel: w652 -> [w869]
        tunnel: w651 -> [w864]
        tunnel: w650 -> [w866]
        tunnel: w649 -> [w841]
        tunnel: w648 -> [w865]
        tunnel: [w865] -> w523
        tunnel: [w863] -> w597
        tunnel: w558 -> [w862]
        tunnel: [w862] -> w557
        tunnel: [w861] -> w542
        tunnel: w546 -> [w861]
        tunnel: [w860] -> w540
        tunnel: w545 -> [w860]
        tunnel: [w859] -> w541
        tunnel: w544 -> [w859]
        tunnel: [w858] -> w535
        tunnel: w539 -> [w857]
        tunnel: [w857] -> w537
        tunnel: [w856] -> w534
        tunnel: [w841] -> w522
        tunnel: w518 -> [w855]
        tunnel: [w855] -> w514
        tunnel: [w854] -> w513
        tunnel: w517 -> [w854]
        tunnel: w516 -> [w853]
        tunnel: [w853] -> w512
        tunnel: w515 -> [w852]
        tunnel: [w852] -> w511
        tunnel: [w851] -> w508
        tunnel: w510 -> [w851]
        tunnel: [w850] -> w507
        tunnel: [w849] -> w506
        tunnel: w488 -> [w848]
        tunnel: w486 -> [w847]
        tunnel: [w846] -> w456
        tunnel: w457 -> [w846]
        tunnel: w411 -> [w845]
        tunnel: [w845] -> w409
        tunnel: w407 -> [w844]
        tunnel: [w844] -> w406
        tunnel: w404 -> [w843]
        tunnel: [w843] -> w403
        tunnel: w402 -> [w837]
        tunnel: [w838] -> w400
        tunnel: [w839] -> w397
        tunnel: w398 -> [w840]
        tunnel: [w842] -> w384
        tunnel: w392 -> [w842]
        tunnel: [w836] -> w372
        tunnel: w373 -> [w836]
        frame #0 {
          n114 = call <vilib>:"IMAQdx Start Acquisition.vi"("error in"=w834, "Session In"=w835) -> ("error out"=w832:errorcluster, "Session Out"=w833:T3)  [unwired: 8 in]
          n115 = call <vilib>:"IMAQdx Start Acquisition.vi"("error in"=w799, "Session In"=w801) -> ("error out"=w798:errorcluster, "Session Out"=w800:T3)  [unwired: 8 in]
          n116 = call <vilib>:"IMAQdx Configure Grab.vi"("error in"=w818, "Session In"=w819) -> ("error out"=w815:errorcluster, "Session Out"=w816:T3)  [unwired: 8 in]
          n117 = call <vilib>:"DAQmx Start Task.vi"("task/channels in"=w829, "error in"=w828) -> ("task out"=w827:refnum<k21>, "error out"=w826:errorcluster)  [unwired: 12 in]
        }
        frame #1 {
          n118 = call <vilib>:"DAQmx Start Task.vi"("task/channels in"=w837, "error in"=w840) -> ("task out"=w838:refnum<k21>, "error out"=w839:errorcluster)  [unwired: 12 in]
          n119 = Tick Count (ms)() -> (millisecond timer value=w863:u32)
          n120 = call <vilib>:"DAQmx Start Task.vi"("task/channels in"=w847, "error in"=w848) -> ("task out"=w850:refnum<k21>, "error out"=w849:errorcluster)  [unwired: 12 in]
          n121 = Tick Count (ms)() -> (millisecond timer value=w858:u32)
          n122 = Tick Count (ms)() -> (millisecond timer value=w856:u32)
          n123 = call <vilib>:"DAQmx Start Task.vi"("task/channels in"=w864, "error in"=w866) -> ("task out"=w868:refnum<k21>, "error out"=w867:errorcluster)  [unwired: 12 in]
        }
      }
      n124 = while {
        tunnel: w507 -> [w751]
        tunnel: [w749] -> w502
        tunnel: w506 -> [w749]
        tunnel: [w751] -> w503
        stop <- w750 stop-if-true
        n125 = local read "Analog Data"() -> (w750:bool)
      }
      n126 = while {
        tunnel: [w926] -> w484
        tunnel: [w912] -> w452
        tunnel: [w930] -> w454
        tunnel: w604 -> [w929]
        tunnel: w605 -> [w928]
        tunnel: w606 -> [w927]
        tunnel: w607 -> [w907]
        shift-right: [w883] -> _
        shift-left: _ -> [w881]
        shift-right: [w878] -> _
        shift-left: u32 0 ("New Lost") -> [w882]
        shift-right: [w880] -> w450
        shift-left: u32[] [] ("NewBuffNum") -> [w879]
        shift-right: [w885] -> w446
        shift-left: u32[] [] ("NewNumLost") -> [w884]
        tunnel: w523 -> [w924]
        tunnel: w597 -> [w916]
        tunnel: w557 -> [w914]
        tunnel: [w912] -> w485
        tunnel: w561 -> [w910]
        tunnel: w560 -> [w909]
        tunnel: [w910] -> w500
        tunnel: [w909] -> w501
        tunnel: w514 -> [w894]
        tunnel: w513 -> [w893]
        tunnel: w512 -> [w892]
        tunnel: w511 -> [w891]
        tunnel: w508 -> [w889]
        tunnel: u32 0 ("y") -> [w886]
        i -> [w887]
        stop <- w921 stop-if-true
        n127 = Multiply(x=w889, y=w887) -> (x*y=w890:dbl)
        n128 = Greater?(x=w887, y=w886) -> (0:→"Whisk Cam":bool)
        n129 = call <vilib>:"IMAQdx Get Image.vi"("Buffer Number Mode (Next)"=IMAQdx_Buffer_Number_Mode."Buffer Number", "error in"=w928, "Buffer Number In"=w887, "Image In"=w927, "Session In"=w929) -> ("error out"=w936:errorcluster, "Buffer Number Out"=w883:u32, "Image Out"=w877:T1, "Session Out"=w926:T3)  [unwired: 3 in]
        "?" <- w877
        n130 = Round Toward -Infinity(1:w890) -> (0:w888:dbl)
        n131 = Tick Count (ms)() -> (millisecond timer value=w917:u32)
        n132 = Index Array(array=w894, index (row)=w888) -> (element=w900:bool[])  [unwired: 1 in]
        n133 = Index Array(array=w893, index (row)=w888) -> (element=w898:bool[])  [unwired: 1 in]
        n134 = Index Array(array=w892, index (row)=w888) -> (element=w896:bool[])  [unwired: 1 in]
        n135 = Index Array(array=w891, index (row)=w888) -> ()  [unwired: 1 in, 1 out]
        n136 = Subtract(x=w917, y=w916) -> (x-y=w920:u32)
        n137 = Add(x=w883, y=w882) -> (x+y=w925:u32)
        n138 = call "IMAQ ImageToArray"("error in (no error)"=w936, "Image"=w877) -> ("error out"=w935:errorcluster, "Image Pixels (U8)"=w934:u8[][])  [unwired: 2 in, 3 out]
        n139 = Multiply(x=w920, y=1.667e-05) -> (x*y=w919:dbl)
        n140 = call <vilib>:"Calculate Frames per Second.vi"("Update Interval (ms)"=u32 2000, "Buffer Number"=w883) -> ("Processed Frames/s"=→"Whisker Cam Fs":dbl)  [unwired: 7 in, 2 out]
        n141 = call "TrackWhiskerDroppedFrames_2P.vi"("NumLost"=w884, "BuffNum"=w879, "Curr Buffer"=w883, "Prev Lost"=w882, "Prev Buffer"=w881) -> ("New Lost"=w878:u32, "NewNumLost"=w885:u32[], "NewBuffNum"=w880:u32[])  [unwired: 4 in]
        "Dropped" <- w878
        n142 = Greater?(x=w900, y=FALSE ("Boolean")) -> (0:w899:bool[])
        n143 = Greater?(x=w898, y=FALSE ("Boolean")) -> (0:w897:bool[])
        n144 = Greater?(x=w896, y=FALSE ("Boolean")) -> (0:w895:bool[])
        n145 = Greater Or Equal?(x=w925, y=w924) -> (x >= y?=w922:bool)
        n146 = Bundle("Time (min)"=w914, w919) -> (→"Time Elapsed (Min)":cluster{"Time (min)":dbl, dbl})  [unwired: 1 in]
        n147 = Write to Binary File(file (use dialog)=w907, data=w934, error in=w935, 5:FALSE ("prepend array or string size? (T)"), 9:T8."little-endian" ("byte order (0:big-endian, network order)")) -> (refnum out=w930:refnum<file>, error out=w912:errorcluster)  [unwired: 1 in, 1 out]
        n148 = local read "Analog Data"() -> (w876:bool)
        n149 = Or Array Elements(Boolean array=w899) -> (logical OR=→"LPad":bool)
        n150 = Or Array Elements(Boolean array=w897) -> (logical OR=→"Auditory":bool)
        n151 = Or Array Elements(Boolean array=w895) -> (logical OR=→"RPad":bool)
        n152 = Unbundle By Name(w912) -> ("status"=w923:bool)
        n153 = Compound Arithmetic op=OR(w876, w923, w922, "stop") -> (w921:bool)
        "Whisker Camera" <- w921
      }
      n154 = while {
        tunnel: [w683] -> w483
        tunnel: [w669] -> w426
        shift-right: [w674] -> _
        shift-left: u32 0 ("Buffer Number Out") -> [w687]
        shift-right: [w686] -> _
        shift-left: u32 0 ("New Lost") -> [w682]
        shift-right: [w685] -> w416
        shift-left: u32[] [] ("NewBuffNum") -> [w673]
        shift-right: [w684] -> w419
        shift-left: u32[] [] ("NewBuffNum") -> [w677]
        tunnel: [w670] -> w482
        tunnel: w456 -> [w671]
        tunnel: [w670] -> w430
        tunnel: w409 -> [w667]
        tunnel: w406 -> [w666]
        tunnel: w403 -> [w665]
        tunnel: w400 -> [w663]
        tunnel: w397 -> [w664]
        tunnel: [w664] -> w396
        tunnel: [w663] -> w395
        tunnel: w384 -> [w662]
        tunnel: u32 0 ("y") -> [w672]
        i -> [w660]
        stop <- w678 stop-if-true
        (unwired) FALSE ("Boolean")
        (unwired) FALSE ("Boolean")
        (unwired) FALSE ("Boolean")
        n155 = Greater?(x=w660, y=w672) -> (0:→"Pupil Cam":bool)
        n156 = call <vilib>:"IMAQdx Get Image.vi"("Buffer Number Mode (Next)"=IMAQdx_Buffer_Number_Mode."Buffer Number", "error in"=w665, "Buffer Number In"=w660, "Image In"=w666, "Session In"=w667) -> ("error out"=w693:errorcluster, "Buffer Number Out"=w674:u32, "Image Out"=w659:T1, "Session Out"=w683:T3)  [unwired: 3 in]
        "?" <- w659
        n157 = Add(x=w674, y=w682) -> (x+y=w681:u32)
        n158 = call "IMAQ ImageToArray"("error in (no error)"=w693, "Image"=w659) -> ("error out"=w692:errorcluster, "Image Pixels (U8)"=w691:u8[][])  [unwired: 2 in, 3 out]
        n159 = call "TrackPupilDroppedFrames_2P.vi"("NumLost"=w677, "BuffNum"=w673, "Curr Buffer"=w674, "Prev Lost"=w682, "Prev Buffer"=w687) -> ("New Lost"=w686:u32, "NewNumLost"=w684:u32[], "NewBuffNum"=w685:u32[])  [unwired: 4 in]
        "Dropped 2" <- w686
        n160 = call <vilib>:"Calculate Frames per Second.vi"("Update Interval (ms)"=u32 2000, "Buffer Number"=w674) -> ("Processed Frames/s"=→"Pupil Cam Fs":dbl)  [unwired: 7 in, 2 out]
        n161 = Greater Or Equal?(x=w681, y=w662) -> (x >= y?=w679:bool)
        n162 = Write to Binary File(file (use dialog)=w671, data=w691, error in=w692, 5:FALSE ("prepend array or string size? (T)"), 9:T8."little-endian" ("byte order (0:big-endian, network order)")) -> (refnum out=w669:refnum<file>, error out=w670:errorcluster)  [unwired: 1 in, 1 out]
        n163 = local read "Analog Data"() -> (w668:bool)
        n164 = local read "stop"() -> (w661:bool)
        n165 = Unbundle By Name(w670) -> ("status"=w680:bool)
        n166 = Compound Arithmetic op=OR(w680, w679, w661, w668) -> (w678:bool)
      }
      n167 = while {
        tunnel: w615 -> [w796]
        tunnel: w616 -> [w795]
        tunnel: w617 -> [w794]
        tunnel: [w793] -> w433
        tunnel: [w777] -> w494
        tunnel: [w792] -> w495
        shift-right: [w785] -> _
        shift-left: w478 -> [w786]
        tunnel: w478 -> [w779]
        tunnel: w522 -> [w778]
        i -> [w780]
        stop <- w783 stop-if-true
        n168 = Greater?(x=w780, y=w779) -> (0:→"Analog":bool)
        n169 = call-poly <vilib>:"DAQmx Read.vi"("task/channels in"=w795, "error in"=w796) -> ("task out"=w792:refnum<k21>, "data"=w790:waveform(dbl)[], "error out"=w784:errorcluster)  [unwired: 11 in]
        n170 = Index Array(array=w790, index=0) -> (element=w788:waveform(dbl))
        n171 = Unbundle By Name(w788) -> ("Y"=w787:dbl[])
        n172 = Array Size(array=w787) -> (size(s)=w782:i32)
        n173 = TDMS Write(0:w794, 5:"Analog Data" ("group name in (Untitled)"), 9:w790, 11:w784) -> (4:w793:refnum<k34>, 15:w777:errorcluster)  [unwired: 2 in, 2 out]
        n174 = Add(x=w782, y=w786) -> (x+y=w785:u32)
        "Analog Samples" <- w785
        n175 = Unbundle By Name(w777) -> ("status"=w775:bool)
        n176 = local read "stop"() -> (w776:bool)
        n177 = Greater Or Equal?(x=w785, y=w778) -> (x >= y?=w774:bool)
        n178 = Compound Arithmetic op=OR(w774, w775, w776) -> (w783:bool)
        "Analog Data" <- w783
      }
      n179 = while {
        tunnel: w542 -> [w761]
        tunnel: w540 -> [w760]
        tunnel: w541 -> [w764]
        tunnel: w537 -> [w763]
        tunnel: [w754] -> w377
        tunnel: [w753] -> w376
        tunnel: [w763] -> w375
        tunnel: w535 -> [w766]
        tunnel: w534 -> [w765]
        i -> [w767]
        stop <- w756 stop-if-true
        n180 = Tick Count (ms)() -> (millisecond timer value=w771:u32)
        n181 = Greater?(x=w766, y=w767) -> (0:→"Behav Cam":bool)
        n182 = Subtract(x=w771, y=w765) -> (x-y=w772:u32)
        n183 = Divide(x=w772, y=u32 1000) -> (x/y=w762:dbl)
        n184 = call "GrabWebCam_2P.vi"("Session In"=w760, "Image In"=w761, "Trial Time"=w762, "AVI Refnum"=w763, "error in"=w764) -> ("Session Out"=w754:T3, "WebCam Img Out"=→"?":T1, "Buffer Number Out"=w758:u32, "error out"=w753:errorcluster)  [unwired: 7 in]
        n185 = call <vilib>:"Calculate Frames per Second.vi"("Update Interval (ms)"=u32 5000, "Buffer Number"=w758) -> ("Processed Frames/s"=→"Behavior Cam Fs":dbl)  [unwired: 7 in, 2 out]
        n186 = local read "Analog Data"() -> (w757:bool)
        n187 = local read "stop"() -> (w755:bool)
        n188 = Unbundle By Name(w753) -> ("status"=w752:bool)
        n189 = Compound Arithmetic op=OR(w752, w755, w757) -> (w756:bool)
      }
      n190 = flat-sequence {
        tunnel: [w728] -> w505
        tunnel: [w727] -> w504
        tunnel: w503 -> [w718]
        tunnel: w502 -> [w726]
        tunnel: w501 -> [w725]
        tunnel: w500 -> [w724]
        tunnel: [w723] -> w499
        tunnel: [w722] -> w498
        tunnel: [w721] -> w497
        tunnel: [w720] -> w496
        tunnel: w495 -> [w719]
        tunnel: w494 -> [w695]
        tunnel: w485 -> [w717]
        tunnel: w484 -> [w716]
        tunnel: w483 -> [w715]
        tunnel: w482 -> [w714]
        tunnel: [w713] -> w455
        tunnel: w454 -> [w713]
        tunnel: w452 -> [w712]
        tunnel: [w712] -> w451
        tunnel: w450 -> [w711]
        tunnel: [w711] -> w449
        tunnel: [w710] -> w447
        tunnel: w446 -> [w710]
        tunnel: w433 -> [w709]
        tunnel: [w709] -> w432
        tunnel: w430 -> [w708]
        tunnel: [w708] -> w429
        tunnel: w426 -> [w707]
        tunnel: [w707] -> w427
        tunnel: w419 -> [w706]
        tunnel: [w706] -> w418
        tunnel: w416 -> [w705]
        tunnel: [w705] -> w415
        tunnel: [w704] -> w410
        tunnel: w396 -> [w703]
        tunnel: w395 -> [w702]
        tunnel: [w701] -> w394
        tunnel: w377 -> [w700]
        tunnel: w376 -> [w698]
        tunnel: w375 -> [w699]
        tunnel: w372 -> [w697]
        tunnel: [w697] -> w371
        tunnel: [w696] -> w366
        tunnel: [w695] -> w364
        tunnel: w505 -> [w748]
        tunnel: w504 -> [w747]
        tunnel: w499 -> [w746]
        tunnel: w498 -> [w745]
        tunnel: w497 -> [w744]
        tunnel: w496 -> [w743]
        tunnel: w455 -> [w742]
        tunnel: [w742] -> w453
        tunnel: w451 -> [w741]
        tunnel: [w741] -> w431
        tunnel: w449 -> [w740]
        tunnel: [w740] -> w448
        tunnel: w447 -> [w739]
        tunnel: [w739] -> w445
        tunnel: w432 -> [w738]
        tunnel: [w738] -> w428
        tunnel: w429 -> [w737]
        tunnel: [w737] -> w360
        tunnel: [w736] -> w361
        tunnel: w427 -> [w736]
        tunnel: w418 -> [w735]
        tunnel: [w735] -> w417
        tunnel: w415 -> [w734]
        tunnel: [w734] -> w414
        tunnel: w410 -> [w733]
        tunnel: w394 -> [w732]
        tunnel: [w731] -> w369
        tunnel: w371 -> [w731]
        tunnel: w366 -> [w730]
        tunnel: [w730] -> w365
        tunnel: [w729] -> _
        tunnel: w364 -> [w729]
        frame #0 {
          n191 = call <vilib>:"DAQmx Stop Task.vi"("task/channels in"=w719, "error in"=w695) -> ("task out"=w721:refnum<k21>, "error out"=w720:errorcluster)  [unwired: 12 in]
          n192 = call <vilib>:"DAQmx Stop Task.vi"("task/channels in"=w718, "error in"=w726) -> ("task out"=w728:refnum<k21>, "error out"=w727:errorcluster)  [unwired: 12 in]
          n193 = call <vilib>:"DAQmx Stop Task.vi"("task/channels in"=w725, "error in"=w724) -> ("task out"=w722:refnum<k21>, "error out"=w723:errorcluster)  [unwired: 12 in]
          n194 = call <vilib>:"IMAQdx Close Camera.vi"("error in"=w698, "Session In"=w700) -> ()  [unwired: 9 in, 1 out]
          n195 = call <vilib>:"DAQmx Stop Task.vi"("task/channels in"=w702, "error in"=w703) -> ("task out"=w704:refnum<k21>, "error out"=w701:errorcluster)  [unwired: 12 in]
          n196 = call "IMAQ AVI2 Close"("error in (no error)"=w698, "AVI Refnum"=w699) -> ("error out"=w696:errorcluster)  [unwired: 9 in]
          n197 = call <vilib>:"IMAQdx Close Camera.vi"("error in"=w714, "Session In"=w715) -> ()  [unwired: 9 in, 1 out]
          n198 = call <vilib>:"IMAQdx Close Camera.vi"("error in"=w717, "Session In"=w716) -> ()  [unwired: 9 in, 1 out]
        }
        frame #1 {
          n199 = call <vilib>:"DAQmx Clear Task.vi"("task in"=w733, "error in"=w732) -> ()  [unwired: 13 in, 1 out]
          n200 = call <vilib>:"DAQmx Clear Task.vi"("task in"=w744, "error in"=w743) -> ()  [unwired: 13 in, 1 out]
          n201 = call <vilib>:"DAQmx Clear Task.vi"("task in"=w745, "error in"=w746) -> ()  [unwired: 13 in, 1 out]
          n202 = call <vilib>:"DAQmx Clear Task.vi"("task in"=w748, "error in"=w747) -> ()  [unwired: 13 in, 1 out]
        }
      }
      n203 = Close File(refnum=w361, error in=w360) -> (path=w359:path, error out=w362:errorcluster)
      n204 = Delete From Array(array=w417, length=1, index=0) -> (array with subset deleted=w412:u32[])  [unwired: 1 out]
      n205 = Delete From Array(array=w445, length=1, index=0) -> (array with subset deleted=w413:u32[])  [unwired: 1 out]
      n206 = Delete From Array(array=w414, length=1, index=0) -> (array with subset deleted=w420:u32[])  [unwired: 1 out]
      n207 = Delete From Array(array=w448, length=1, index=0) -> (array with subset deleted=w644:u32[])  [unwired: 1 out]
      n208 = Close File(refnum=w453, error in=w431) -> (path=w621:path, error out=w622:errorcluster)
      n209 = Move(source path=w359, error in=w362, 10:"Target Path") -> (error out=w363:errorcluster)  [unwired: 2 in, 2 out]
      n210 = Move(source path=w369, error in=w365, 10:"Target Path") -> (error out=w543:errorcluster)  [unwired: 2 in, 2 out]
      n211 = Move(source path=w621, error in=w622, 10:"Target Path") -> (error out=w624:errorcluster)  [unwired: 2 in, 2 out]
      n212 = Build Array(w420, w412) -> (w422:u32[][])
      n213 = Build Array(w644, w413) -> (w421:u32[][])
      n214 = call <vilib>:"Simple Error Handler.vi"("error in (no error)"=w363) -> ()  [unwired: 1 in, 8 out]
      n215 = Array To Spreadsheet String(delimiter (Tab)=",", array=w420, 3:"%d" ("format string")) -> (spreadsheet string=w442:string)
      n216 = Array To Spreadsheet String(delimiter (Tab)=",", array=w412, 3:"%d" ("format string")) -> (spreadsheet string=w443:string)
      n217 = Array To Spreadsheet String(delimiter (Tab)=",", array=w644, 3:"%d" ("format string")) -> (spreadsheet string=w637:string)
      n218 = Array To Spreadsheet String(delimiter (Tab)=",", array=w413, 3:"%d" ("format string")) -> (spreadsheet string=w638:string)
      n219 = Transpose 2D Array(2D array=w422) -> (transposed array=w444:u32[][])
      n220 = Transpose 2D Array(2D array=w421) -> (transposed array=w643:u32[][])
      n221 = call <vilib>:"Simple Error Handler.vi"("error in (no error)"=w624) -> ()  [unwired: 1 in, 8 out]
      n222 = call <vilib>:"Simple Error Handler.vi"("error in (no error)"=w543) -> ()  [unwired: 1 in, 8 out]
      n223 = call <vilib>:"Trim Whitespace.vi"("string"=w442) -> ("trimmed string"=w368:string)  [unwired: 1 in]
      n224 = call <vilib>:"Trim Whitespace.vi"("string"=w637) -> ("trimmed string"=w521:string)  [unwired: 1 in]
      n225 = call <vilib>:"Trim Whitespace.vi"("string"=w443) -> ("trimmed string"=w367:string)  [unwired: 1 in]
      n226 = call <vilib>:"Trim Whitespace.vi"("string"=w638) -> ("trimmed string"=w639:string)  [unwired: 1 in]
      n227 = Number To Decimal String(number=w444) -> ()  [unwired: 1 in, 1 out]
      n228 = Number To Decimal String(number=w643) -> ()  [unwired: 1 in, 1 out]
      n229 = Build Array(w521, w639, w368, w367) -> (w640:string[])
      n230 = TDMS Set Properties(5:w640, 7:string[] ["WhiskerCam_DroppedFrameIndex", "WhiskerCam_NumberDropped", "PupilCam_DroppedFrameIndex", "PupilCam_NumberDropped"] ("channel name(s) in (Untitled)"), 8:w431, 11:w428) -> (0:w635:errorcluster, 3:w636:refnum<k34>)  [unwired: 2 in, 2 out]
      n231 = TDMS Close(8:w635, 11:w636) -> (0:w620:errorcluster, 3:w625:path)
      n232 = Path To String(path=w625) -> (string=w520:string)
      n233 = Concatenate Strings(w520, "_index" ("string")) -> (w626:string)
      n234 = TDMS Defragment(4:w620, 7:w625) -> (0:w628:errorcluster)
      n235 = String To Path(string=w626) -> (path=w627:path)
      n236 = Move(source path=w625, error in=w628, 10:"Target Path") -> (error out=w623:errorcluster)  [unwired: 2 in, 2 out]
      n237 = Move(source path=w627, error in=w628, 10:"Target Path") -> (error out=w519:errorcluster)  [unwired: 2 in, 2 out]
      n238 = call <vilib>:"Simple Error Handler.vi"("error in (no error)"=w519) -> ()  [unwired: 1 in, 8 out]
      n239 = call <vilib>:"Simple Error Handler.vi"("error in (no error)"=w623) -> ()  [unwired: 1 in, 8 out]
    }
    frame #4 {
      "Complete" <- TRUE ("Data Acquisition - Complete")
    }
  }
